vi "RubikTurnFSM.vi"(1 "Turn":T1) -> ()   [LabVIEW 2017]
uses:
  Controls/RubikMoves.ctl
  Controls/ServoRelAngleControl.ctl
  Controls/ServoEnumControl.ctl
  8eb4d94e-5852-4223-b3f1-68aace851966.vi
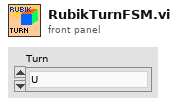
[diagram p1: front panel]
types:
  T1 = typedef "RubikMoves.ctl" = enum16{"U", "U'", "F", "F'", "D", "D'", "B", "B'", "L", "L'", "R", "R'"}
  T2 = typedef "ServoRelAngleControl.ctl" = enum16{"-90°", "+90°"}
  T3 = typedef "ServoEnumControl.ctl" = enum16{"Left Servo", "Front Servo", "Right Servo"}
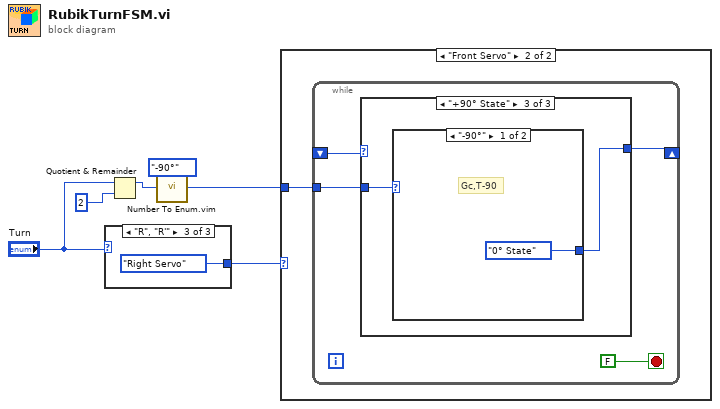
[diagram p0: block diagram]
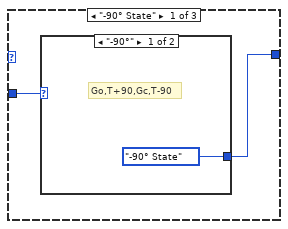
[diagram p3: hidden frame]
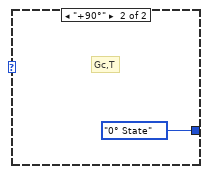
[diagram p4: hidden frame]
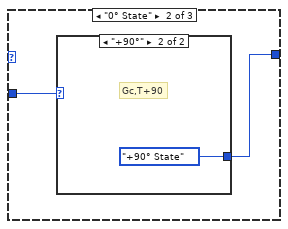
[diagram p5: hidden frame]
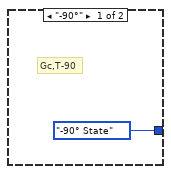
[diagram p6: hidden frame]
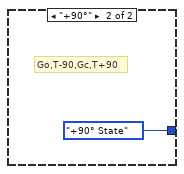
[diagram p7: hidden frame]
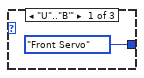
[diagram p8: hidden frame]
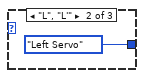
[diagram p9: hidden frame]
diagram:
  n1 = case shown="\"R\", \"R'\"" "Turn" {
    tunnel: [ServoEnumControl."Front Servo" ("Servo Enum") ServoEnumControl."Left Servo" ("Servo Enum") ServoEnumControl."Right Servo" ("Servo Enum")] -> w6
    frame "U".."B'" {
    }
    frame "L", "L'" {
    }
    frame "R", "R'" {
    }
  }
  n2 = Quotient & Remainder(x="Turn", y=2) -> (x-y*floor(x/y)=w3:i32)  [unwired: 1 out]
  n3 = call "Number To Enum.vim"("number"=w3, "enum type"=ServoRelAngleControl."-90°" ("Turn by")) -> ("number as enum"=w1:T2)
  n4 = case shown="\"Front Servo\"" w6 {
    tunnel: w1 -> [_ w10]
    frame "Left Servo", Default {
    }
    frame "Front Servo" {
      n5 = while {
        shift-right: [w13] -> _
        shift-left: _ -> [w14]
        tunnel: w10 -> [w11]
        stop <- FALSE stop-if-true
        n6 = case shown="\"+90° State\"" w14 {
          tunnel: [w16 w20 w24] -> w13
          tunnel: w11 -> [w15 w19 w23]
          frame "-90° State" {
            n7 = case shown="\"-90°\"" w15 {
              tunnel: [enum16{"-90° State", "0° State", "+90° State"}."-90° State" ("Enum 2") enum16{"-90° State", "0° State", "+90° State"}."0° State" ("Enum 2")] -> w16
              frame "-90°" {
                # "Go,T+90,Gc,T-90"
              }
              frame "+90°" {
                # "Gc,T"
              }
            }
          }
          frame "0° State" {
            n8 = case shown="\"+90°\"" w19 {
              tunnel: [enum16{"-90° State", "0° State", "+90° State"}."-90° State" ("Enum 2") enum16{"-90° State", "0° State", "+90° State"}."+90° State" ("Enum 2")] -> w20
              frame "-90°" {
                # "Gc,T-90"
              }
              frame "+90°" {
                # "Gc,T+90"
              }
            }
          }
          frame "+90° State" {
            n9 = case shown="\"-90°\"" w23 {
              tunnel: [enum16{"-90° State", "0° State", "+90° State"}."0° State" ("Enum 2") enum16{"-90° State", "0° State", "+90° State"}."+90° State" ("Enum 2")] -> w24
              frame "-90°" {
                # "Gc,T-90"
              }
              frame "+90°" {
                # "Go,T-90,Gc,T+90"
              }
            }
          }
        }
      }
    }
  }
